vi "List Test Node MAC.vi"(8 "error in (no error)":errorcluster, 11 "Edit Test Node Model in":refnum<class "Edit Test Node Model.lvclass">) -> (0 "error out":errorcluster, 3 "Edit Test Node Model out":refnum<class "Edit Test Node Model.lvclass">)   [LabVIEW 2013, in "Edit Test Node Model.lvlib" / "Edit Test Node Model.lvclass"]
uses:
  Edit Test Node Model.lvclass
  Edit Test Node Model.lvclass/Edit Test Node Model.ctl
  <vilib>/ActorFrameworkMVC/View Observer/View Registry/View Registry.lvclass/View Registry.ctl
  Edit Test Node Model Messages/Abstract Edit Test Node List Msg/Abstract Edit Test Node List Msg.lvclass
  <vilib>/ActorFrameworkMVC/View Observer/Data Message/Data Message.lvclass
  <vilib>/ActorFrameworkMVC/View Observer/View Registry/View Registry.lvclass
  Common/ZDAQ/ZDAQ.lvlib
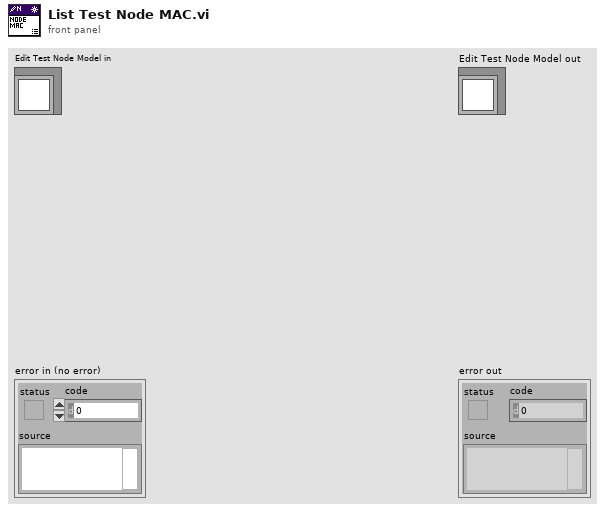
[diagram p1: front panel]
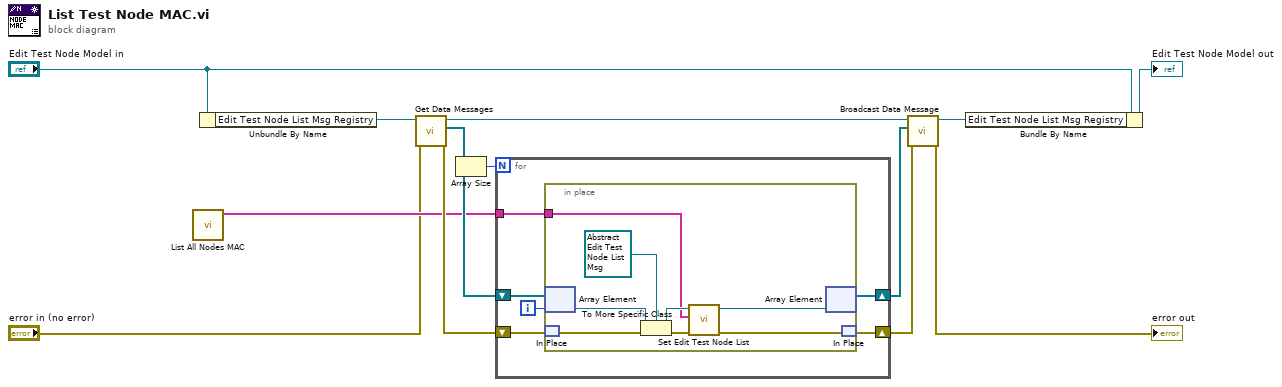
[diagram p0: block diagram]
diagram:
  n1 = call "List All Nodes MAC.vi"() -> ("Nodes MAC List"=w5:string[])  [unwired: 10 in, 1 out]
  n2 = Unbundle By Name("Edit Test Node Model in") -> ("Edit Test Node List Msg Registry"=w13:refnum<class "View Registry.lvclass">)
  n3 = call <vilib>:"Get Data Messages.vi"("error in (no error)"="error in (no error)", "View Registry in"=w13) -> ("error out"=w9:errorcluster, "Data Messages"=w10:refnum<class "Data Message.lvclass">[], "View Registry out"=w12:refnum<class "View Registry.lvclass">)  [unwired: 7 in]
  n4 = Array Size(array=w10) -> (size(s)=w11:i32)
  n5 = for {
    N: w11 -> [_]
    shift-right: [w18] -> w8
    shift-left: w10 -> [w19]
    shift-right: [w15] -> w7
    shift-left: w9 -> [w17]
    tunnel: w5 -> [w16]
    i -> [w14]
    n6 = in-place {
      in-place-border: w16 -> [w20]
      n7 = in-place-array #1(w19, w14) -> (w25:refnum<class "Data Message.lvclass">)
      n8 = in-place-match #2(w17) -> (w27:errorcluster)
      n9 = To More Specific Class(target class=refnum<class "Abstract Edit Test Node List Msg.lvclass"> refnum ("Edit Test Node Model.lvlib:Abstract Edit Test Node List Msg.lvclass"), reference=w25, error in=w27) -> (specific class reference=w21:refnum<class "Abstract Edit Test Node List Msg.lvclass">, error out=w24:errorcluster)
      n10 = call "Set Edit Test Node List.vi"("error in (no error)"=w24, "Edit Test Node List"=w20, "Abstract Edit Test Node List Msg in"=w21) -> ("error out"=w23:errorcluster, "Abstract Edit Test Node List Msg out"=w22:refnum<class "Abstract Edit Test Node List Msg.lvclass">)  [unwired: 7 in]
      n11 = in-place-array #1(w22) -> (w18:refnum<class "Data Message.lvclass">[])  [unwired: 1 out]
      n12 = in-place-match #2(w23) -> (w15:errorcluster)
    }
  }
  n13 = call <vilib>:"Broadcast Data Message.vi"("error in (no error)"=w7, "Data Messages"=w8, "View Registry in"=w12) -> ("error out"=→"error out":errorcluster, "View Registry out"=w6:refnum<class "View Registry.lvclass">)  [unwired: 7 in]
  n14 = Bundle By Name(cluster="Edit Test Node Model in", "Edit Test Node List Msg Registry"=w6) -> (→"Edit Test Node Model out":refnum<class "Edit Test Node Model.lvclass">)
